vi "TDMS - File Viewer (NXG Style).vi"(8 "error in":errorcluster, 11 "file in":path) -> (0 "error out":errorcluster={"status"=TRUE, "code"=118, "source"="TDMS Open in TDMS - File Viewer with Flat Layout.vi"}, 3 "file out":path)   [LabVIEW 2019, in "NI_TDMS File Viewer.lvlib"]
doc: "Opens the .tdms file specified in the <B>file path</B> input and presents the file data in the TDMS File Viewer dialog box."
uses:
  NI_TDMS File Viewer.lvlib
  <vilib>/Utility/error.llb/DialogType.ctl
  Global VI for Localized Text.vi
panel:
  in  "File Tree":string[](tree)
  out "Property Table":string[][](table)
  in  "All":bool
  in  "Samples":i64=100000 min=-1 step=1
  in  "Start index":i64 min=0 step=1
  out "Waveform Graph":waveform(dbl)[](graph)
  in  "Value Table":i32(listbox)=-1
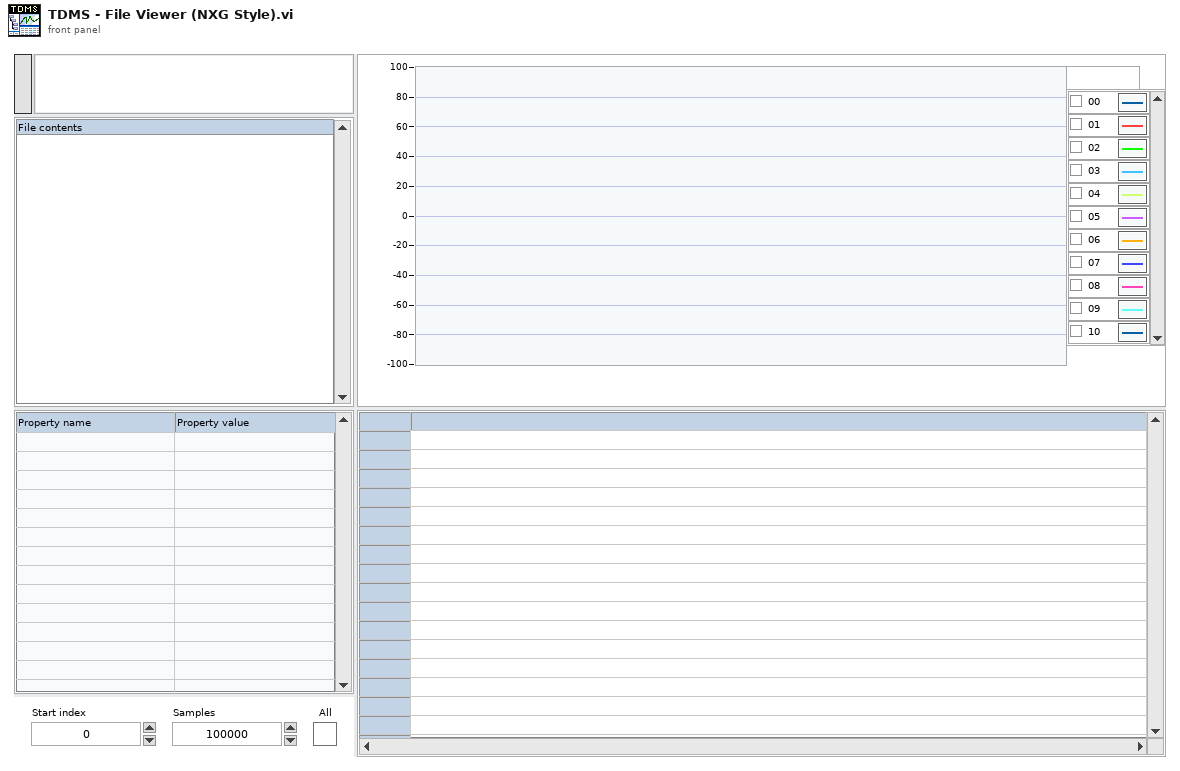
[diagram p1: front panel]
types:
  T1 = enum16{"open", "open or create", "create or replace", "create", "open (read-only)"}
  T2 = cluster{"All":bool, "Start index":i64, "Samples":i64}
  T3 = enum8{"Enabled", "Disabled", "Disabled and Grayed Out"}
  T4 = typedef "eventvkey.ctl" = enum16{"ASCII", "Enter", "Return", "Shift", "Ctrl", "Alt", "Cmd", "Opt", "Caps", "NumLock", "Clear", "Break", "Up", "Down", "Left", "Right", "Insert", "Delete", "Home", "End", "PageUp", "PageDown", "Escape", "Help", "Pause", "ScrollLock", "F1", "F2", "F3", "F4", "F5", "F6", "F7", "F8", "F9", "F10", "F11", "F12", "F13", "F14", "F15", "F16", "F17", "F18", "F19", "F20", "F21", "F22", "F23", "F24", "Play", "VolumeUp", "VolumeDown", "Mute", "Two Byte Char"}
  T5 = typedef "LVPoint32TypeDef.ctl" = cluster{"Horizontal":i32, "Vertical":i32}
  T6 = typedef "NI_TDMS File Viewer.lvlib/Table Components.ctl" = cluster{"column headers":string[], "row headers":string[], "values":string[][]}
  T7 = typedef "DialogType.ctl" = u16
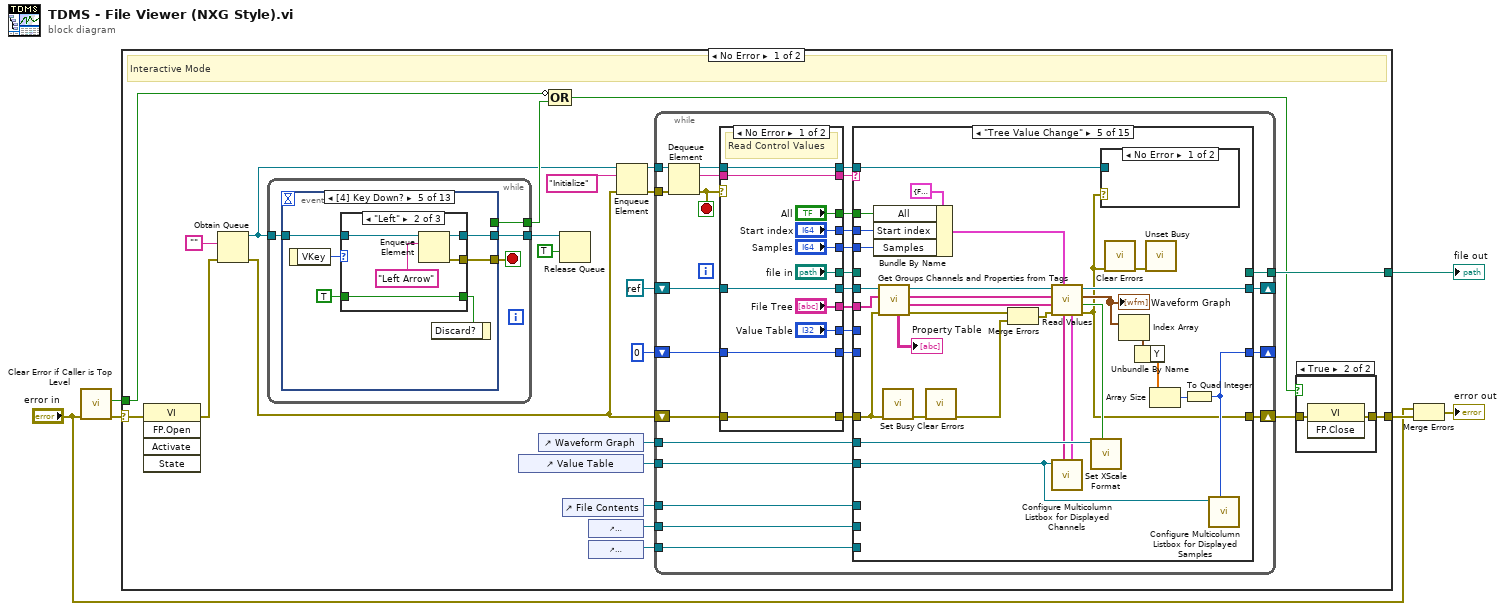
[diagram p0: block diagram]
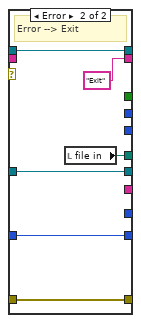
[diagram p3: hidden frame]
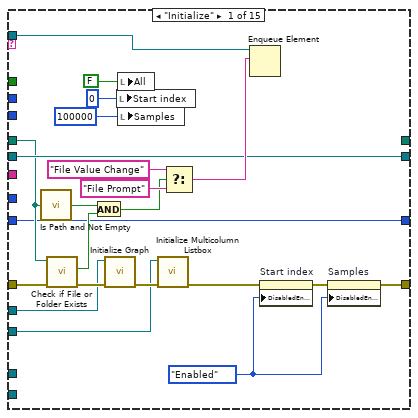
[diagram p4: hidden frame]
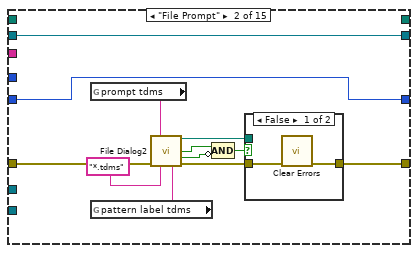
[diagram p5: hidden frame]
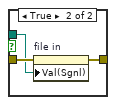
[diagram p6: hidden frame]
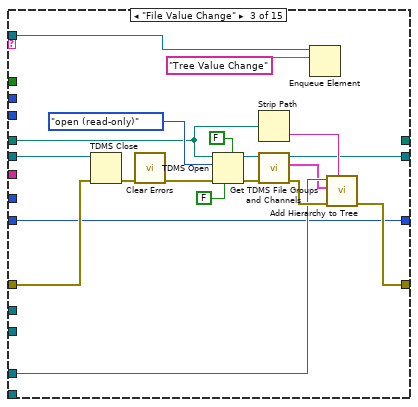
[diagram p7: hidden frame]
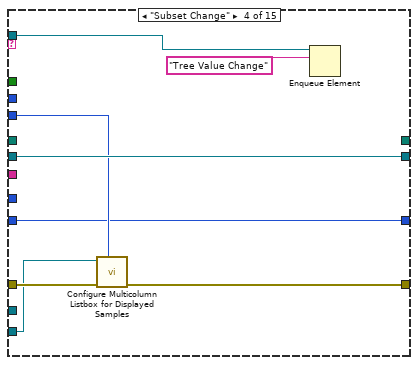
[diagram p8: hidden frame]
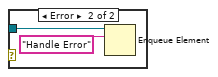
[diagram p9: hidden frame]
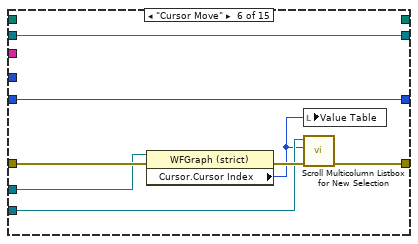
[diagram p10: hidden frame]
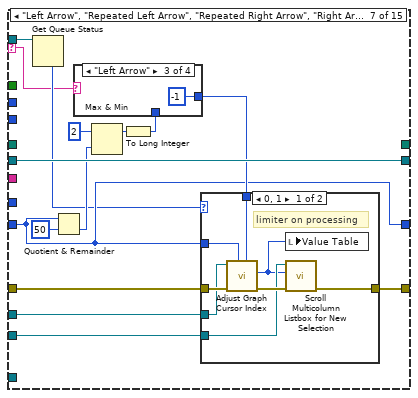
[diagram p11: hidden frame]
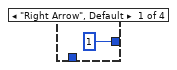
[diagram p13: hidden frame]
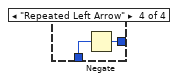
[diagram p15: hidden frame]
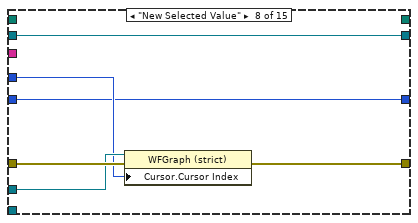
[diagram p16: hidden frame]
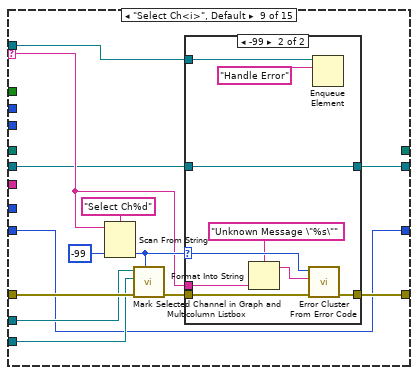
[diagram p17: hidden frame]
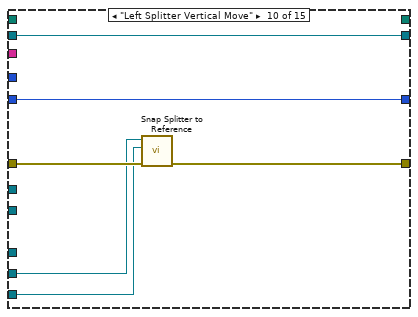
[diagram p19: hidden frame]
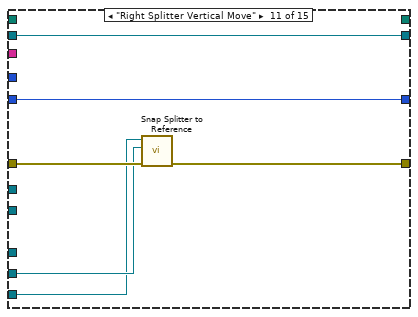
[diagram p20: hidden frame]
diagram:
  n1 = call "Clear Error if Caller is Top Level.vi"("error in"="error in") -> ("error out"=w6:errorcluster, "top level"=w1:bool)  [unwired: 9 in]
  n2 = case shown="No Error" w6 {
    selector: w6 -> [w9 w393]
    tunnel: [w20 _] -> w2
    tunnel: [w28 w393] -> w5
    tunnel: w1 -> [w16 _]
    frame No Error {
      # "Interactive Mode"
      n3 = invoke class="VI" method="FP.Open"(error in=w9) -> (error out=w8:errorcluster)  [unwired: 4 in, 4 out]
      n4 = Obtain Queue(element data type="", error in (no error)=w8) -> (queue out=w7:refnum<queue>, error out=w10:errorcluster)  [unwired: 3 in, 1 out]
      n5 = while {
        tunnel: [w287] -> w19
        tunnel: w7 -> [w286]
        tunnel: [w285] -> w14
        stop <- w288 stop-if-true
        n6 = event shown="[4] Key Down?" {
          selector: _ -> [_ _ _ _ _ _ _ _ _ _ _ _ _]
          dyn-events: _ -> [_ _ _ _ _ _ _ _ _ _ _ _ _]
          timeout: _ -> [_ _ _ _ _ _ _ _ _ _ _ _ _]
          tunnel: [w290 w299 w307 w322 w326 w343 w360 w364 w368 w377 w381 w385 w389] -> w288
          tunnel: [_ _ _ _ _ _ _ _ _ _ _ _ w391] -> w287
          tunnel: w286 -> [w291 w300 w308 w323 w327 w344 w361 w365 w369 w378 w382 w386 w390]
          tunnel: [w289 w298 w306 w321 w325 w342 w359 w363 w367 w376 w380 w384 w388] -> w285
          event "Start index", "Samples": Value Change {
            n7 = event-data() -> ()  [unwired: 1 in, 1 out]
            n8 = local read "Start index"() -> (w296:i64)
            n9 = local read "Samples"() -> (w295:i64)
            n10 = Less Than 0?(x=w295) -> (x < 0?=w294:bool)
            n11 = Equal To 0?(x=w296) -> (x = 0?=w293:bool)
            n12 = And(x=w294, y=w293) -> (x .and. y?=w292:bool)
            n13 = local write "All"(w292) -> ()
            n14 = Enqueue Element(queue=w291, element="Subset Change" ("CHM or HLP filename (lvdialog.chm)")) -> (queue out=w289:refnum<queue>, error out=w290:errorcluster)  [unwired: 2 in, 1 out]
          }
          event "All": Value Change {
            n15 = event-data() -> ("NewVal"=w302:bool)  [unwired: 1 in]
            n16 = Select(t=T3."Disabled and Grayed Out" ("Disabled"), s=w302, f=T3."Enabled" ("Disabled")) -> (s? t:f=w301:T3)
            n17 = property on="Start index" class="DigNum (strict)"("DisabledEnum"=w301) -> ()  [unwired: 2 in, 2 out]
            n18 = property on="Samples" class="DigNum (strict)"("DisabledEnum"=w301) -> ()  [unwired: 2 in, 2 out]
            n19 = Enqueue Element(queue=w300, element="Subset Change" ("CHM or HLP filename (lvdialog.chm)")) -> (queue out=w298:refnum<queue>, error out=w299:errorcluster)  [unwired: 2 in, 1 out]
          }
          event "file in": Value Change {
            n20 = event-data() -> ("OldVal"=w309:path, "NewVal"=w313:path)  [unwired: 1 in]
            n21 = call <vilib>:"Is Path and Not Empty.vi"("path"=w313) -> ("Is Path and Not Empty?"=w312:bool)  [unwired: 4 in]
            n22 = call <vilib>:"Check if File or Folder Exists.vi"("path"=w313) -> ("file or folder exists?"=w311:bool)  [unwired: 8 in, 2 out]
            n23 = And(x=w311, y=w312) -> (x .and. y?=w310:bool)
            n24 = case shown="False" w310 {
              tunnel: "File Value Change" ("CHM or HLP filename (lvdialog.chm)") -> [_ w320]
              tunnel: w309 -> [w316 _]
              tunnel: w308 -> [w315 w319]
              tunnel: [_ w318] -> w307
              tunnel: [w315 w317] -> w306
              frame False {
                n25 = local write "file in"(w316) -> ()
              }
              frame True {
                n26 = Enqueue Element(queue=w319, element=w320) -> (queue out=w317:refnum<queue>, error out=w318:errorcluster)  [unwired: 2 in, 1 out]
              }
            }
          }
          event "File Tree": Value Change {
            n27 = event-data() -> ()  [unwired: 1 in, 1 out]
            n28 = Enqueue Element(queue=w323, element="Tree Value Change" ("CHM or HLP filename (lvdialog.chm)")) -> (queue out=w321:refnum<queue>, error out=w322:errorcluster)  [unwired: 2 in, 1 out]
          }
          event Key Down? {
            n29 = event-data() -> ("VKey"=w330:T4)  [unwired: 1 in]
            n30 = case shown="\"Left\"" w330 {
              tunnel: [_ w335 w340] -> w328
              tunnel: TRUE ("Discard?") -> [_ w335 w340]
              tunnel: w327 -> [w331 w334 w339]
              tunnel: [_ w333 w338] -> w326
              tunnel: [w331 w332 w337] -> w325
              frame Default {
              }
              frame "Left" {
                n31 = Enqueue Element(queue=w334, element="Left Arrow" ("CHM or HLP filename (lvdialog.chm)")) -> (queue out=w332:refnum<queue>, error out=w333:errorcluster)  [unwired: 2 in, 1 out]
              }
              frame "Right" {
                n32 = Enqueue Element(queue=w339, element="Right Arrow" ("CHM or HLP filename (lvdialog.chm)")) -> (queue out=w337:refnum<queue>, error out=w338:errorcluster)  [unwired: 2 in, 1 out]
              }
            }
            n33 = event-data("Discard?"=w328) -> ()  [unwired: 1 in, 1 out]
          }
          event event type 5.0.x8000000b {
            n34 = event-data() -> ("VKey"=w347:T4)  [unwired: 1 in]
            n35 = case shown="\"Right\"" w347 {
              tunnel: [_ w352 w357] -> w346
              tunnel: TRUE ("abort (F)") -> [_ w352 w357]
              tunnel: w344 -> [w348 w351 w356]
              tunnel: [_ w350 w355] -> w343
              tunnel: [w348 w349 w354] -> w342
              frame Default {
              }
              frame "Left" {
                n36 = Enqueue Element(queue=w351, element="Repeated Left Arrow" ("CHM or HLP filename (lvdialog.chm)")) -> (queue out=w349:refnum<queue>, error out=w350:errorcluster)  [unwired: 2 in, 1 out]
              }
              frame "Right" {
                n37 = Enqueue Element(queue=w356, element="Repeated Right Arrow" ("CHM or HLP filename (lvdialog.chm)")) -> (queue out=w354:refnum<queue>, error out=w355:errorcluster)  [unwired: 2 in, 1 out]
              }
            }
            n38 = event-data("Discard?"=w346) -> ()  [unwired: 1 in, 1 out]
          }
          event "Waveform Graph": Cursor Move {
            n39 = event-data() -> ()  [unwired: 1 in, 1 out]
            n40 = Enqueue Element(queue=w361, element="Cursor Move" ("CHM or HLP filename (lvdialog.chm)")) -> (queue out=w359:refnum<queue>, error out=w360:errorcluster)  [unwired: 2 in, 1 out]
          }
          event "Value Table": Value Change {
            n41 = event-data() -> ()  [unwired: 1 in, 1 out]
            n42 = Enqueue Element(queue=w365, element="New Selected Value" ("CHM or HLP filename (lvdialog.chm)")) -> (queue out=w363:refnum<queue>, error out=w364:errorcluster)  [unwired: 2 in, 1 out]
          }
          event "Value Table": Double Click {
            n43 = event-data() -> ("CtlRef"=w375:refnum<vi>, "Coords"=w370:T5)  [unwired: 1 in]
            n44 = call "Coordinates to Multicolumn Listbox Column.vi"("Coords"=w370, "MulticolumnListbox in"=w375) -> ("Column"=w373:i32)  [unwired: 9 in]
            n45 = Format Into String(format string="%d", initial string="Select Ch" ("CHM or HLP filename (lvdialog.chm)"), w373) -> (resulting string=w371:string)  [unwired: 1 in, 1 out]
            n46 = Enqueue Element(queue=w369, element=w371) -> (queue out=w367:refnum<queue>, error out=w368:errorcluster)  [unwired: 2 in, 1 out]
          }
          event Mouse Leave; Mouse Up {
            n47 = event-data() -> ()  [unwired: 1 in, 1 out]
            n48 = Enqueue Element(queue=w378, element="Left Splitter Vertical Move" ("CHM or HLP filename (lvdialog.chm)")) -> (queue out=w376:refnum<queue>, error out=w377:errorcluster)  [unwired: 2 in, 1 out]
          }
          event Mouse Leave; Mouse Up {
            n49 = event-data() -> ()  [unwired: 1 in, 1 out]
            n50 = Enqueue Element(queue=w382, element="Right Splitter Vertical Move" ("CHM or HLP filename (lvdialog.chm)")) -> (queue out=w380:refnum<queue>, error out=w381:errorcluster)  [unwired: 2 in, 1 out]
          }
          event Pane Size {
            n51 = event-data() -> ()  [unwired: 1 in, 1 out]
            n52 = Enqueue Element(queue=w386, element="Graph Resize" ("CHM or HLP filename (lvdialog.chm)")) -> (queue out=w384:refnum<queue>, error out=w385:errorcluster)  [unwired: 2 in, 1 out]
          }
          event Panel Close? {
            w389 = errorcluster {"status"=TRUE, "code"=0, "source"=""}  # Stop
            w391 = TRUE ("Discard?")
            n53 = event-data() -> ()  [unwired: 1 in, 1 out]
            n54 = Enqueue Element(queue=w390, element="Exit" ("CHM or HLP filename (lvdialog.chm)")) -> (queue out=w388:refnum<queue>)  [unwired: 2 in, 2 out]
            n55 = event-data("Discard?"=w391) -> ()  [unwired: 1 in, 1 out]
          }
        }
      }
      n56 = control-ref of="Value Table"() -> (w26:refnum<vi>)
      n57 = control-ref of="Waveform Graph"() -> (w23:refnum<vi>)
      n58 = Compound Arithmetic op=OR(invert w16, w19) -> (w18:bool)
      n59 = Release Queue(queue=w14, force destroy? (F)=TRUE) -> ()  [unwired: 1 in, 3 out]
      n60 = control-ref of="File Contents"() -> (w25:refnum<vi>)
      n61 = control-ref of="Splitter:ValueTableTop"() -> (w22:refnum<vi>)
      n62 = control-ref of="Splitter:PropTableTop"() -> (w21:refnum<vi>)
      n63 = Enqueue Element(queue=w7, element="Initialize" ("CHM or HLP filename (lvdialog.chm)"), error in (no error)=w10) -> (queue out=w15:refnum<queue>, error out=w12:errorcluster)  [unwired: 1 in, 1 out]
      n64 = while {
        tunnel: w15 -> [w57]
        shift-right: [w46] -> _
        shift-left: refnum<k0> refnum -> [w47]
        shift-right: [w58] -> w29
        shift-left: w10 -> [w59]
        tunnel: w26 -> [w45]
        tunnel: w25 -> [w44]
        tunnel: w23 -> [w42]
        tunnel: w22 -> [w41]
        tunnel: w21 -> [w40]
        tunnel: [w39] -> w20
        shift-right: [w36] -> _
        shift-left: i64 0 -> [w37]
        tunnel: w12 -> [w33]
        stop <- w56 stop-if-true
        n65 = Dequeue Element(queue=w57, error in (no error)=w33) -> (queue out=w35:refnum<queue>, element=w54:string, error out=w56:errorcluster)  [unwired: 1 in, 1 out]
        n66 = case shown="No Error" w56 {
          tunnel: [w70 "Exit" ("element")] -> w55
          tunnel: w54 -> [w70 _]
          tunnel: ["file in" w74] -> w53
          tunnel: ["File Tree" _] -> w52
          tunnel: ["Samples" _] -> w51
          tunnel: ["Start index" _] -> w50
          tunnel: ["All" _] -> w49
          tunnel: [w64 w75] -> w48
          tunnel: w47 -> [w64 w75]
          tunnel: [w71 w77] -> w60
          tunnel: w59 -> [w71 w77]
          tunnel: ["Value Table" _] -> w43
          tunnel: [w62 w73] -> w38
          tunnel: w37 -> [w62 w73]
          tunnel: [w61 w72] -> w34
          tunnel: w35 -> [w61 w72]
          frame No Error {
            # "Read Control Values"
          }
          frame Error {
            # "Error --> Exit"
            n67 = local read "file in"() -> (w74:path)
          }
        }
        n68 = case shown="\"Tree Value Change\"" w55 {
          selector: w55 -> [_ _ _ _ _ _ w184 _ w222 _ _ _ _ _ _]
          tunnel: w53 -> [w93 _ w118 _ _ _ _ _ _ _ _ _ _ w275 _]
          tunnel: w52 -> [_ _ _ _ w152 _ _ _ _ _ _ _ _ _ _]
          tunnel: w51 -> [_ _ _ w138 w165 _ _ _ _ _ _ _ _ _ _]
          tunnel: w50 -> [_ _ _ _ w166 _ _ _ _ _ _ _ _ _ _]
          tunnel: w49 -> [_ _ _ _ w167 _ _ _ _ _ _ _ _ _ _]
          tunnel: w45 -> [w80 _ _ w139 w155 w178 w194 _ w225 _ _ _ _ _ _]
          tunnel: w48 -> [w94 w103 w124 w141 w169 w180 w196 w216 w219 w246 w252 w259 w264 w277 w280]
          tunnel: [w94 w103 w120 w141 w168 w180 w196 w216 w220 w246 w252 w259 w264 refnum<k0> refnum w280] -> w46
          tunnel: w60 -> [w99 w111 w134 w143 w150 w183 w198 w217 w231 w248 w253 w262 w266 w278 w283]
          tunnel: w44 -> [_ _ w123 _ _ _ _ _ _ _ _ _ _ _ _]
          tunnel: [w96 w109 w130 w142 w151 w181 w197 w218 w229 w247 w254 w260 w265 w278 w284] -> w58
          tunnel: w43 -> [_ _ _ _ _ _ _ w214 _ _ _ _ _ _ _]
          tunnel: w42 -> [w92 _ _ _ w163 w179 w195 w215 w226 _ _ w258 _ _ _]
          tunnel: w41 -> [_ _ _ _ _ _ _ _ _ w245 w251 w257 _ _ _]
          tunnel: w40 -> [_ _ _ _ _ _ _ _ _ w244 w250 w256 _ _ _]
          tunnel: [_ _ _ _ _ _ _ _ _ _ _ _ _ w275 _] -> w39
          tunnel: w38 -> [w82 w100 w119 w137 _ w176 w192 w213 w223 w243 w249 w255 w263 w274 w279]
          tunnel: [w82 w100 w119 w137 w154 w176 w192 w213 w223 w243 w249 w255 w263 w274 w279] -> w36
          tunnel: w34 -> [w79 _ w117 w136 w144 _ w186 _ w221 _ _ _ _ _ _]
          frame "Initialize" {
            w83 = T3."Enabled" ("Disabled")
            n69 = call <vilib>:"Is Path and Not Empty.vi"("path"=w93) -> ("Is Path and Not Empty?"=w89:bool)  [unwired: 4 in]
            n70 = call <vilib>:"Check if File or Folder Exists.vi"("error in (no error)"=w99, "path"=w93) -> ("error out"=w98:errorcluster, "file or folder exists?"=w88:bool)  [unwired: 7 in, 1 out]
            n71 = And(x=w89, y=w88) -> (x .and. y?=w87:bool)
            n72 = call "Initialize Graph.vi"("error in"=w98, "WaveformGraph"=w92) -> ("error out"=w81:errorcluster)  [unwired: 9 in]
            n73 = local write "Start index"(i64 0 ("Start index")) -> ()
            n74 = local write "All"(FALSE ("All")) -> ()
            n75 = local write "Samples"(i64 100000 ("Samples")) -> ()
            n76 = call "Initialize Multicolumn Listbox.vi"("error in"=w81, "MulticolumnListbox"=w80) -> ("error out"=w78:errorcluster)  [unwired: 9 in]
            n77 = Select(t="File Value Change" ("CHM or HLP filename (lvdialog.chm)"), s=w87, f="File Prompt" ("CHM or HLP filename (lvdialog.chm)")) -> (s? t:f=w95:string)
            n78 = Enqueue Element(queue=w79, element=w95) -> ()  [unwired: 2 in, 3 out]
            n79 = property on="Start index" class="DigNum (strict)"(error in=w78, "DisabledEnum"=w83) -> (error out=w97:errorcluster)  [unwired: 1 in, 1 out]
            n80 = property on="Samples" class="DigNum (strict)"(error in=w97, "DisabledEnum"=w83) -> (error out=w96:errorcluster)  [unwired: 1 in, 1 out]
          }
          frame "File Prompt" {
            n81 = global read "Global VI for Localized Text.vi" "prompt tdms"() -> (w107:string)
            n82 = global read "Global VI for Localized Text.vi" "pattern label tdms"() -> (w106:string)
            n83 = call "File Dialog2"("prompt"=w107, "error in"=w111, "pattern (all files)"="*.tdms", "pattern label"=w106) -> ("selected path"=w104:path, "exists"=w102:bool, "cancelled"=w101:bool, "error out"=w110:errorcluster)  [unwired: 3 in, 5 out]
            n84 = Compound Arithmetic op=AND(w102, invert w101) -> (w105:bool)
            n85 = case shown="False" w105 {
              tunnel: w110 -> [w113 w116]
              tunnel: [w112 w115] -> w109
              tunnel: w104 -> [_ w114]
              frame False {
                n86 = call <vilib>:"Clear Errors.vi"("error in (no error)"=w113) -> ("error out"=w112:errorcluster)  [unwired: 5 in, 1 out]
              }
              frame True {
                n87 = property on="file in" class="Path"(error in=w116, "Val(Sgnl)"=w114) -> (error out=w115:errorcluster)  [unwired: 1 in, 1 out]
              }
            }
          }
          frame "File Value Change" {
            n88 = TDMS Close(8:w134, 11:w124) -> (0:w133:errorcluster)  [unwired: 1 out]
            n89 = call <vilib>:"Clear Errors.vi"("error in (no error)"=w133) -> ("error out"=w132:errorcluster)  [unwired: 5 in, 1 out]
            n90 = TDMS Open(5:FALSE ("create index file? (T)"), 6:FALSE ("disable buffering (T)"), 8:w132, 10:T1."open (read-only)" ("operation"), 11:w118) -> (0:w135:errorcluster, 3:w125:refnum<k34>)  [unwired: 2 in]
            n91 = Strip Path(path=w118) -> (name=w122:string)  [unwired: 1 out]
            n92 = call "Get TDMS File Groups and Channels.vi"("error in"=w135, "TDMS ref in"=w125) -> ("error out"=w131:errorcluster, "file contents"=w121:cluster{string, string[]}[], "TDMS ref out"=w120:refnum<k34>)  [unwired: 7 in]
            n93 = Enqueue Element(queue=w117, element="Tree Value Change" ("CHM or HLP filename (lvdialog.chm)")) -> ()  [unwired: 2 in, 3 out]
            n94 = call "Add Hierarchy to Tree.vi"("file name"=w122, "error in"=w131, "file contents"=w121, "file tree refnum"=w123) -> ("error out"=w130:errorcluster)  [unwired: 7 in]
          }
          frame "Subset Change" {
            n95 = call "Configure Multicolumn Listbox for Displayed Samples.vi"("Samples"=w138, "error in"=w143, "MulticolumnListbox in"=w139) -> ("error out"=w142:errorcluster)  [unwired: 7 in, 1 out]
            n96 = Enqueue Element(queue=w136, element="Tree Value Change") -> ()  [unwired: 2 in, 3 out]
          }
          frame "Tree Value Change" {
            n97 = Bundle By Name(cluster=T2 {"All"=FALSE, "Start index"=0, "Samples"=0}, "All"=w167, "Start index"=w166, "Samples"=w165) -> (w164:T2)
            n98 = call "Get Groups Channels and Properties from Tags.vi"("error in"=w150, "File Tree"=w152, "tdms file in"=w169) -> ("error out"=w147:errorcluster, "channel names out"=w172:string[], "group names out"=w171:string[], "tdms file out"=w170:refnum<k34>, "property table"=→"Property Table":string[][])  [unwired: 2 in]
            n99 = call <vilib>:"Set Busy.vi"("error in (no error)"=w150) -> ("error out"=w153:errorcluster)  [unwired: 9 in, 1 out]
            n100 = call <vilib>:"Clear Errors.vi"("error in (no error)"=w153) -> ("error out"=w149:errorcluster)  [unwired: 5 in, 1 out]
            n101 = Merge Errors(w147, w149) -> (w148:errorcluster)
            n102 = call "Read Values.vi"("read subset"=w164, "error in"=w148, "channel names"=w172, "group names"=w171, "tdms file"=w170) -> ("error out"=w151:errorcluster, "waveform timestamps = 0"=w158:bool, "waveform values"=w159:waveform(dbl)[], "tdms file out"=w168:refnum<k34>, "table values"=w162:T6, "widest value strings"=w160:string[])  [unwired: 1 in]
            "Waveform Graph" <- w159
            n103 = call "Configure Multicolumn Listbox for Displayed Channels.vi"("table values"=w162, "widest value strings"=w160, "MulticolumnListbox in"=w155) -> ()  [unwired: 7 in]
            n104 = call "Set XScale Format.vi"("timestamp eq 0"=w158, "Waveform Graph"=w163) -> ()  [unwired: 8 in]
            n105 = case shown="No Error" w151 {
              tunnel: w144 -> [_ w174]
              frame No Error {
              }
              frame Error {
                n106 = Enqueue Element(queue=w174, element="Handle Error") -> ()  [unwired: 2 in, 3 out]
              }
            }
            n107 = call <vilib>:"Clear Errors.vi"("error in (no error)"=w151) -> ("error out"=w173:errorcluster)  [unwired: 5 in, 1 out]
            n108 = Index Array(array=w159) -> (element=w156:waveform(dbl))  [unwired: 1 in]
            n109 = Unbundle By Name(w156) -> ("Y"=w157:dbl[])
            n110 = call <vilib>:"Unset Busy.vi"("error in (no error)"=w173) -> ()  [unwired: 10 in, 1 out]
            n111 = Array Size(array=w157) -> (size(s)=w146:i32)
            n112 = To Quad Integer(1:w146) -> (0:w154:i64)
            n113 = call "Configure Multicolumn Listbox for Displayed Samples.vi"("Samples"=w154, "MulticolumnListbox in"=w155) -> ()  [unwired: 8 in, 2 out]
          }
          frame "Cursor Move" {
            n114 = property class="WFGraph (strict)"(reference=w179, error in=w183) -> (error out=w182:errorcluster, "Cursor.Cursor Index"=w177:i32)  [unwired: 1 out]
            n115 = local write "Value Table"(w177) -> ()
            n116 = call "Scroll Multicolumn Listbox for New Selection.vi"("error in"=w182, "new index"=w177, "MulticolumnListbox"=w178) -> ("error out"=w181:errorcluster)  [unwired: 8 in]
          }
          frame "Left Arrow", "Repeated Left Arrow", "Repeated Right Arrow", "Right Arrow" {
            n117 = Get Queue Status(queue=w186) -> (# elements in queue=w185:i32)  [unwired: 2 in, 7 out]
            n118 = Quotient & Remainder(x=w192, y=i64 50) -> (floor(x/y)=w190:i64)  [unwired: 1 out]
            n119 = Max & Min(x=i64 2, y=w190) -> (max(x,y)=w188:i64)  [unwired: 1 out]
            n120 = To Long Integer(number=w188) -> (32bit integer=w187:i32)
            n121 = case shown="\"Left Arrow\"" w184 {
              tunnel: [1 w209 -1 w211] -> w193
              tunnel: w187 -> [_ w209 _ w212]
              frame "Right Arrow", Default {
              }
              frame "Repeated Right Arrow" {
              }
              frame "Left Arrow" {
              }
              frame "Repeated Left Arrow" {
                n122 = Negate(x=w212) -> (-x=w211:i32)
              }
            }
            n123 = case shown="0, 1" w185 {
              tunnel: w195 -> [w203 _]
              tunnel: w198 -> [w206 w207]
              tunnel: w194 -> [w202 _]
              tunnel: [w204 w207] -> w197
              tunnel: w193 -> [w200 _]
              tunnel: w192 -> [w199 _]
              frame 0, 1 {
                # "limiter on processing"
                n124 = call "Adjust Graph Cursor Index.vi"("index adjustment"=w200, "Plot 0 samples"=w199, "error in"=w206, "WaveformGraph in"=w203) -> ("error out"=w205:errorcluster, "adjusted index"=w201:i32)  [unwired: 6 in]
                n125 = local write "Value Table"(w201) -> ()
                n126 = call "Scroll Multicolumn Listbox for New Selection.vi"("error in"=w205, "new index"=w201, "MulticolumnListbox"=w202) -> ("error out"=w204:errorcluster)  [unwired: 8 in]
              }
              frame Default {
                # "When message backlog is high, we don't execute time consuming code to adjust graph cursor position and value table"
              }
            }
          }
          frame "New Selected Value" {
            n127 = property class="WFGraph (strict)"(reference=w215, error in=w217, "Cursor.Cursor Index"=w214) -> (error out=w218:errorcluster)  [unwired: 1 out]
          }
          frame "Select Ch<i>", Default {
            n128 = Scan From String(format string="Select Ch%d", input string=w222, default 1=-99 ("default value 1")) -> (output 1=w224:i32)  [unwired: 2 in, 3 out]
            n129 = call "Mark Selected Channel in Graph and Multicolumn Listbox.vi"("selected channel"=w224, "error in"=w231, "Value Table"=w225, "WaveformGraph"=w226) -> ("error out"=w230:errorcluster)  [unwired: 7 in]
            n130 = case shown="-99" w224 {
              selector: w224 -> [_ w240]
              tunnel: w230 -> [w233 w242]
              tunnel: [w233 w241] -> w229
              tunnel: w222 -> [_ w238]
              tunnel: w221 -> [_ w235]
              tunnel: [w232 w234] -> w220
              tunnel: w219 -> [w232 w234]
              frame Default {
              }
              frame -99 {
                n131 = Format Into String(format string="Unknown Message \"%s\"", w238) -> (resulting string=w237:string)  [unwired: 2 in, 1 out]
                n132 = call <vilib>:"Error Cluster From Error Code.vi"("error in (no error)"=w242, "error message (\"\")"=w237, "error code (0)"=w240) -> ("error out"=w241:errorcluster)  [unwired: 6 in]
                n133 = Enqueue Element(queue=w235, element="Handle Error") -> ()  [unwired: 2 in, 3 out]
              }
            }
          }
          frame "Left Splitter Vertical Move" {
            n134 = call "Snap Splitter to Reference.vi"("error in"=w248, "splitter on move"=w244, "reference splitter"=w245) -> ("error out"=w247:errorcluster)  [unwired: 8 in]
          }
          frame "Right Splitter Vertical Move" {
            n135 = call "Snap Splitter to Reference.vi"("error in"=w253, "splitter on move"=w251, "reference splitter"=w250) -> ("error out"=w254:errorcluster)  [unwired: 8 in]
          }
          frame "Graph Resize" {
            n136 = call "Set Waveform Graph LegNumRows.vi"("error in"=w262, "WaveformGraph"=w258) -> ("error out"=w261:errorcluster)  [unwired: 9 in]
            n137 = call "Snap Splitter to Reference.vi"("error in"=w261, "splitter on move"=w256, "reference splitter"=w257) -> ("error out"=w260:errorcluster)  [unwired: 8 in]
          }
          frame "Handle Error" {
            n138 = case shown="Error .." w266 {
              selector: w266 -> [w267 w272]
              tunnel: [w267 w271] -> w265
              frame No Error {
                # "No Trouble Found"
              }
              frame Error {
                w270 = T7 4 items=["no dialog", "OK message", "continue or stop message", "OK message + warnings", "continue/stop + warnings"] ("type of dialog (OK msg:1)")
                # "Report errors"
                n139 = Unbundle By Name(w272) -> ("code"=w269:i32, "source"=w268:string)
                n140 = call <vilib>:"Simple Error Handler.vi"("error code (no error:0)"=w269, "error source (\" \")"=w268, "type of dialog (OK msg:1)"=w270, "error in (no error)"=w272) -> ("error out"=w273:errorcluster)  [unwired: 1 in, 4 out]
                n141 = call <vilib>:"Clear Errors.vi"("error in (no error)"=w273) -> ("error out"=w271:errorcluster)  [unwired: 5 in, 1 out]
              }
            }
          }
          frame "", "Exit" {
            n142 = TDMS Close(8:w278, 11:w277) -> ()  [unwired: 2 out]
          }
          frame "Launch Help" {
            n143 = call "Launch Help.vi"("error in"=w283, "CHM or HLP filename (lvdialog.chm)"="lvdialog.chm", "HTML filename"="tdms_file_viewer_db.html") -> ("error out"=w284:errorcluster)  [unwired: 4 out]
          }
        }
      }
      n144 = case shown="True" w18 {
        tunnel: w29 -> [w30 w32]
        tunnel: [w30 w31] -> w28
        frame False {
        }
        frame True {
          n145 = invoke class="VI" method="FP.Close"(error in=w32) -> (error out=w31:errorcluster)  [unwired: 2 in, 2 out]
        }
      }
    }
    frame Error {
      # "If TDMS File Viewer running as subVI, input error immediately returns."
    }
  }
  "file out" <- w2
  n146 = Merge Errors("error in", w5) -> (→"error out":errorcluster)
